vi "parse_response.vi"(8 "error in":errorcluster, 9 "handle_out":u64, 10 "response_len_out":i32, 11 "status_out":u32) -> (0 "error out":errorcluster, 3 "response":string)   [LabVIEW 2020, in "reqwest.lvclass"]
uses:
  reqwest.lvclass
  reqwest.lvclass/reqwest.ctl
  shared-library/reqwest-labview.lvlib
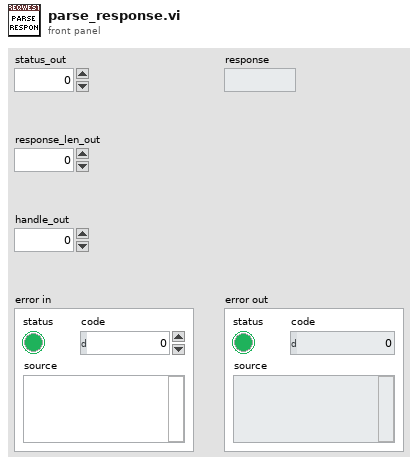
[diagram p1: front panel]
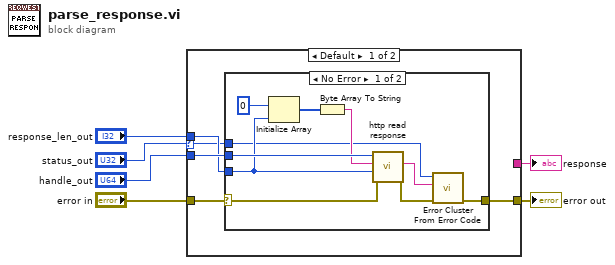
[diagram p0: block diagram]
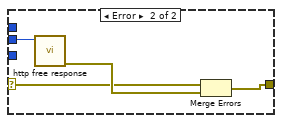
[diagram p2: hidden frame]
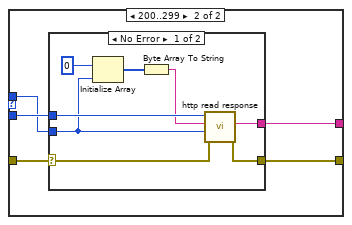
[diagram p3: hidden frame]
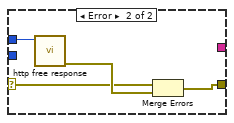
[diagram p4: hidden frame]
diagram:
  n1 = case shown="Default" "status_out" {
    selector: "status_out" -> [w8 _]
    tunnel: "handle_out" -> [w10 w30]
    tunnel: "response_len_out" -> [w9 w29]
    tunnel: [_ w28] -> w1
    tunnel: "error in" -> [w11 w27]
    tunnel: [w7 w26] -> w2
    frame Default {
      n2 = case shown="No Error" w11 {
        selector: w11 -> [w20 w23]
        tunnel: w10 -> [w21 w25]
        tunnel: w9 -> [w17 _]
        tunnel: [w12 w22] -> w7
        tunnel: w8 -> [w15 _]
        frame No Error {
          n3 = Initialize Array(u8 0, w17) -> (w19:u8[])
          n4 = Byte Array To String(unsigned byte array=w19) -> (string=w16:string)
          n5 = call "http read response.vi"("error in (no error)"=w20, "buf_len"=w17, "buf_ptr"=w16, "handle"=w21) -> ("error out"=w13:errorcluster, "buf_ptr out"=w14:string)  [unwired: 4 in, 2 out]
          n6 = call <vilib>:"Error Cluster From Error Code.vi"("error in (no error)"=w13, "error message (\"\")"=w14, "error code (0)"=w15) -> ("error out"=w12:errorcluster)  [unwired: 6 in]
        }
        frame Error {
          n7 = call "http free response.vi"("handle"=w25) -> ("error out"=w24:errorcluster)  [unwired: 8 in, 2 out]
          n8 = Merge Errors(w23, w24) -> (w22:errorcluster)
        }
      }
    }
    frame 200..299 {
      n9 = case shown="No Error" w27 {
        selector: w27 -> [w36 w40]
        tunnel: w30 -> [w38 w42]
        tunnel: w29 -> [w33 _]
        tunnel: [w37 _] -> w28
        tunnel: [w31 w39] -> w26
        frame No Error {
          n10 = Initialize Array(u8 0, w33) -> (w35:u8[])
          n11 = Byte Array To String(unsigned byte array=w35) -> (string=w32:string)
          n12 = call "http read response.vi"("error in (no error)"=w36, "buf_len"=w33, "buf_ptr"=w32, "handle"=w38) -> ("error out"=w31:errorcluster, "buf_ptr out"=w37:string)  [unwired: 4 in, 2 out]
        }
        frame Error {
          n13 = call "http free response.vi"("handle"=w42) -> ("error out"=w41:errorcluster)  [unwired: 8 in, 2 out]
          n14 = Merge Errors(w40, w41) -> (w39:errorcluster)
        }
      }
    }
  }
  "error out" <- w2
  "response" <- w1
